vi "LIA Example Host.vi"() -> ()   [LabVIEW 2017]
uses:
  lib/host/Public/pll settings.ctl
  lib/host/Public/lock-in settings.ctl
  lib/interface/Interface/LIA Host Interface.lvclass
  lib/host/Lock-In Amplifier Example Host.lvlib
  lib/shared/Lock-In Amplifier Example Shared.lvlib
panel:
  out "Waveform Graph":cluster{"f0":dbl, "df":dbl, "magnitude":dbl[]}[](graph)
  in  "app.quit":bool
  in  "lock-in.boxcar length 0":u32=2048 caption="Boxar Length"
  in  "app.tab 0":enum32{"Lock-In", "PLL", "Output"}(tab)
  in  "lock-in.manual carrier 0":dbl=10000000.0 caption="Carrier" format="%#_6p"
  in  "lock-in.decimation 0":i32=2048 caption="Decimation" min=8 max=8192
  in  "lock-in.source 0":enum16{"AI 0", "AI 1", "AI 2", "AI 3"}(ring)=enum."AI 1" caption="Channel"
  in  "lock-in.carrier 0":T1(ring)=enum."PLL 0" caption="Carrier Source"
  in  "pll.source 0":enum16{"AI 0", "AI 1", "AI 2", "AI 3"}(ring) caption="Source"
  in  "pll.q frequency 0":dbl=10000000.0 caption="Q Frequency" format="%#_6p"
  in  "pll.reset 0":bool
  in  "ao.noise 3":dbl caption="A0 3 Noise" min=0.0 max=1.0 format="%#_6p"
  in  "ao.level 3":dbl=0.5 caption="A0 3 Level" format="%#_6pV"
  in  "ao.frequency 3":dbl=10000000.0 caption="AO 3 Frequency" format="%#.9p"
  in  "ao.frequency 0":dbl=10000000.0 caption="AO 0 Frequency" format="%#.9p"
  in  "ao.level 0":dbl=0.5 caption="AO 0 Level" format="%#_6pV"
  in  "rio device":tag="10.2.224.40" caption="Resource"
  in  "lock-in.reset boxar 0":bool
  out "lock-in.deviation 1":dbl=1.9775797561733533e-07 caption="Deviation" format="%#_6p"
  out "lock-in.amplitude 0":dbl=8.221341747482856e-05 caption="Result" format="%#_6p"
  in  "lock-in.boxcar lookback 0":i32=1024 caption="Windows to Average"
  out "Result":cluster{"mean":dbl, "trace":dbl}(graph)={"mean"=8.221341747482856e-05, "trace"=8.36741779633565e-05}
  # "NI Lock-In Amplifier Reference Example"
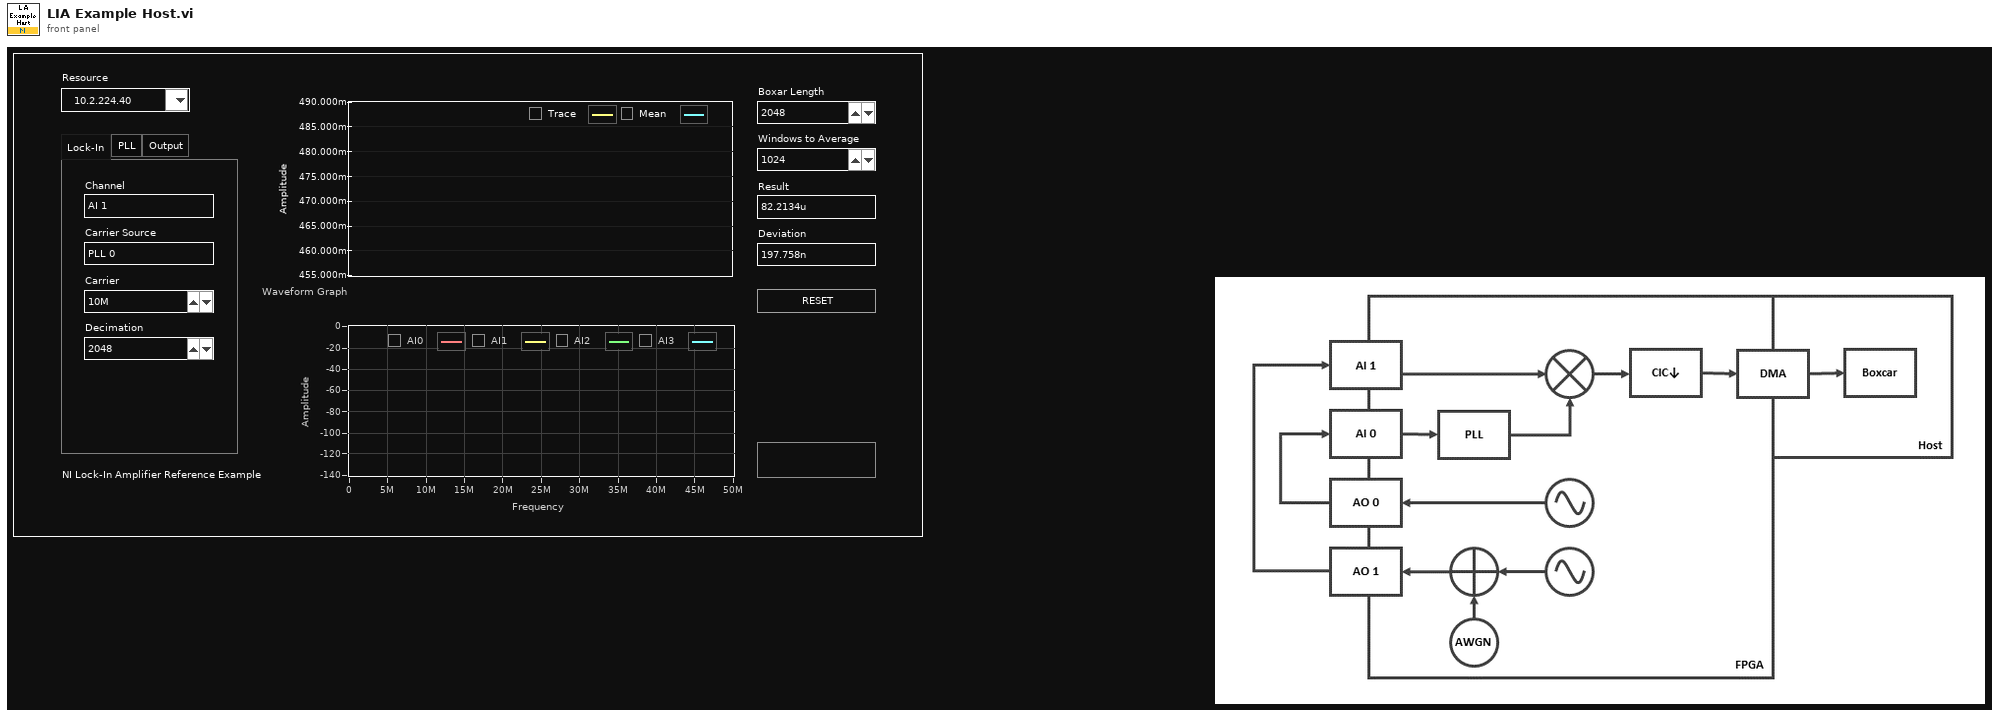
[diagram p1: front panel]
types:
  T1 = enum16{"Manual 0", "Manual 1", "Manual 2", "Manual 3", "PLL 0", "PLL 1"}
  T2 = typedef "Lock-In Amplifier Example Host.lvlib/lock-in settings.ctl" = cluster{"decimation":i32, "source":i32, "carrier source":i32, "carrier":dbl}
  T3 = typedef "Lock-In Amplifier Example Host.lvlib/pll settings.ctl" = cluster{"source":i32, "q frequency":dbl}
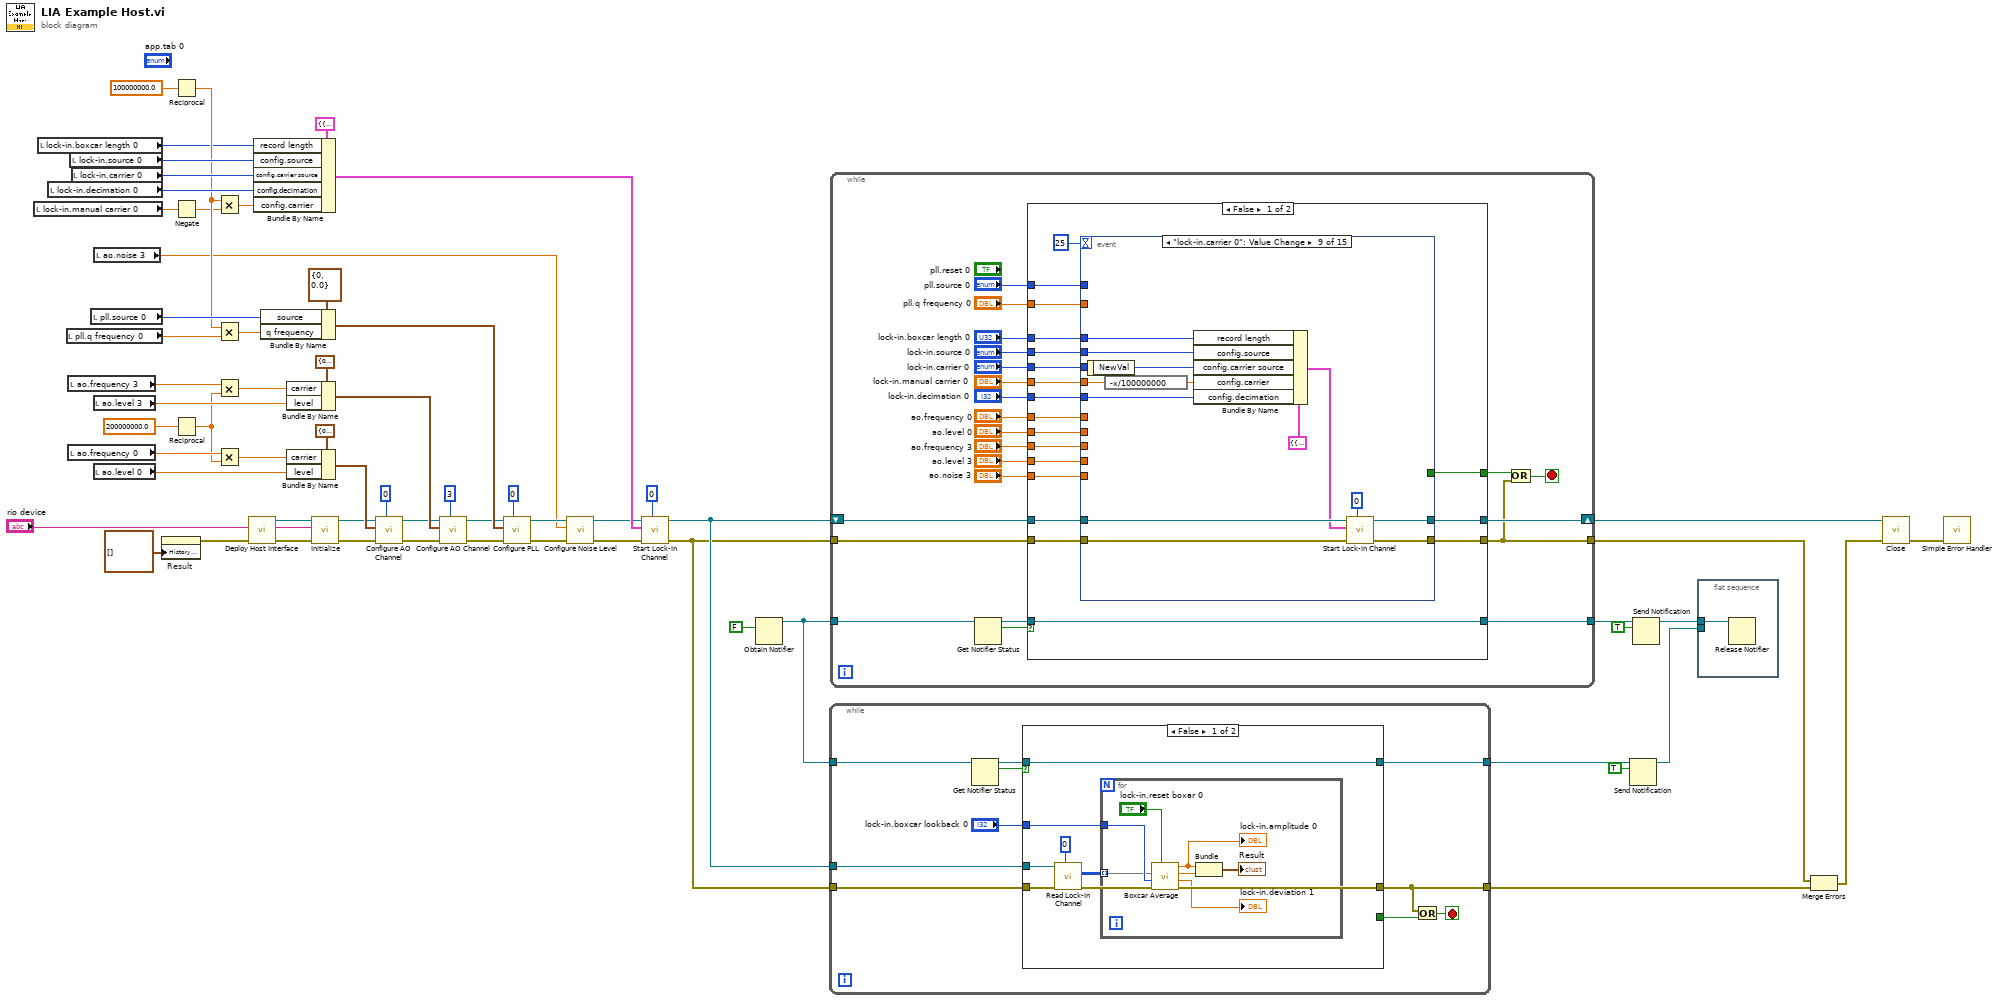
[diagram p0: block diagram]
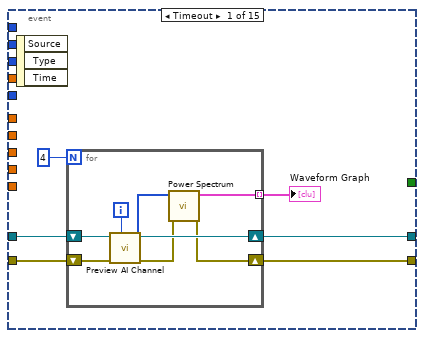
[diagram p2: hidden frame]
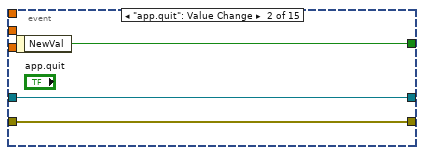
[diagram p3: hidden frame]
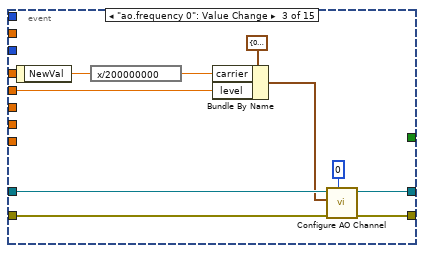
[diagram p4: hidden frame]
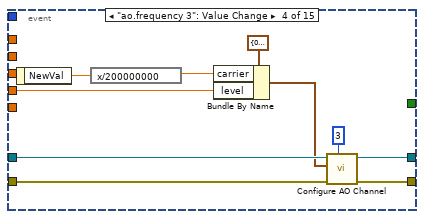
[diagram p5: hidden frame]
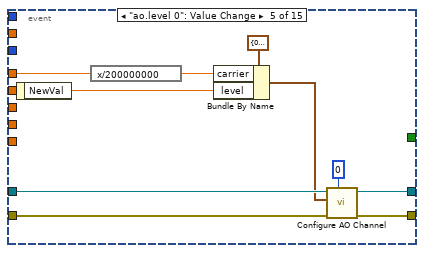
[diagram p6: hidden frame]
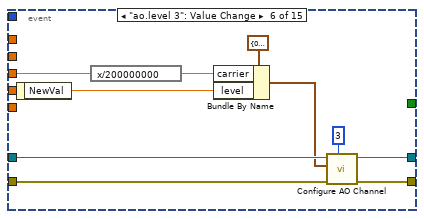
[diagram p7: hidden frame]
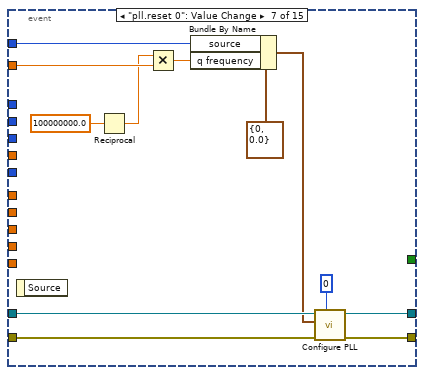
[diagram p8: hidden frame]
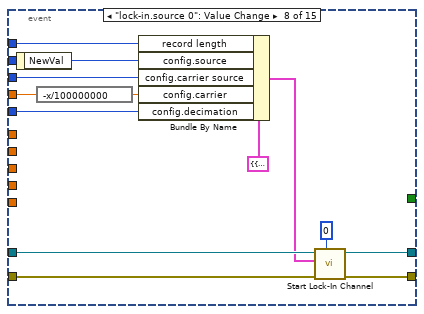
[diagram p9: hidden frame]
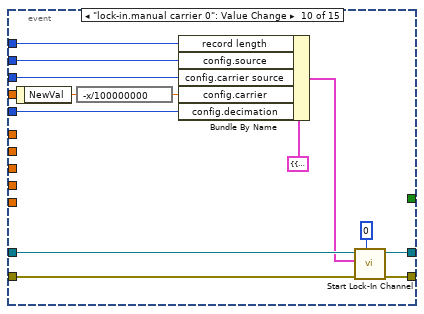
[diagram p10: hidden frame]
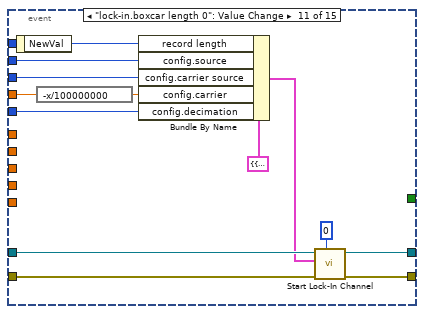
[diagram p11: hidden frame]
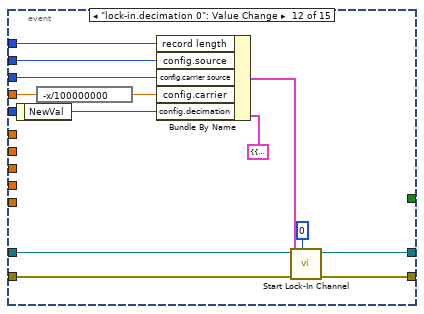
[diagram p12: hidden frame]
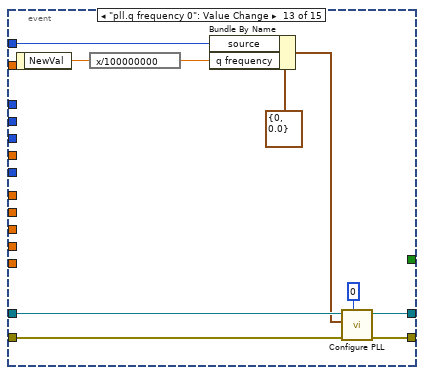
[diagram p13: hidden frame]
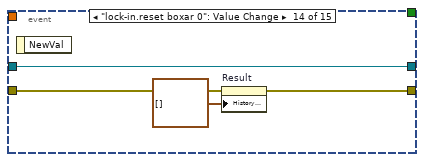
[diagram p14: hidden frame]
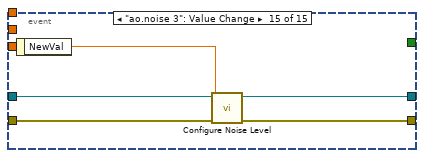
[diagram p15: hidden frame]
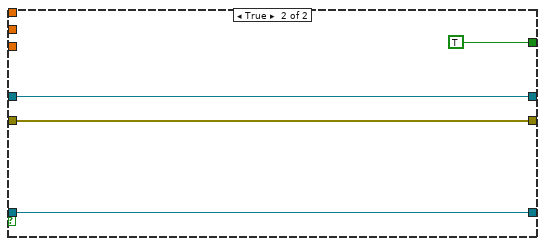
[diagram p16: hidden frame]
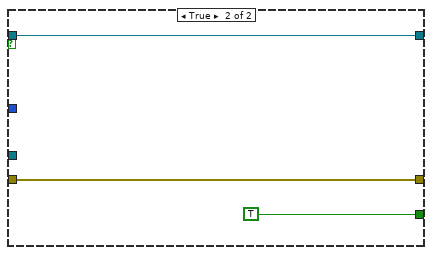
[diagram p17: hidden frame]
diagram:
  n1 = local read "lock-in.manual carrier 0"() -> (w50:dbl)
  n2 = local read "lock-in.boxcar length 0"() -> (w13:u32)
  n3 = local read "lock-in.decimation 0"() -> (w53:i32)
  n4 = local read "pll.q frequency 0"() -> (w55:dbl)
  n5 = local read "ao.frequency 3"() -> (w47:dbl)
  n6 = local read "ao.frequency 0"() -> (w44:dbl)
  n7 = local read "lock-in.source 0"() -> (w64:enum16{"AI 0", "AI 1", "AI 2", "AI 3"})
  n8 = local read "lock-in.carrier 0"() -> (w63:T1)
  n9 = local read "pll.source 0"() -> (w61:enum16{"AI 0", "AI 1", "AI 2", "AI 3"})
  n10 = local read "ao.level 3"() -> (w59:dbl)
  n11 = local read "ao.level 0"() -> (w58:dbl)
  n12 = local read "ao.noise 3"() -> (w2:dbl)
  n13 = property on="Result" class="WFChart (strict)"("History Data"=cluster{"mean":dbl, "trace":dbl}[] []) -> (error out=w8:errorcluster)  [unwired: 2 in, 1 out]
  n14 = Reciprocal(x=100000000.0) -> (1/x=w51:dbl)
  n15 = Negate(x=w50) -> (-x=w49:dbl)
  n16 = Reciprocal(x=200000000.0) -> (1/x=w43:dbl)
  n17 = Multiply(x=w51, y=w49) -> (x*y=w52:dbl)
  n18 = Multiply(x=w51, y=w55) -> (x*y=w56:dbl)
  n19 = Multiply(x=w47, y=w43) -> (x*y=w48:dbl)
  n20 = Multiply(x=w44, y=w43) -> (x*y=w45:dbl)
  n21 = call "Deploy Host Interface.vi"("error in"=w8, "resource"="rio device") -> ("error out"=w9:errorcluster, "resource out"=w10:string, "lia host interface"=w11:refnum<class "LIA Host Interface.lvclass">)  [unwired: 7 in]
  n22 = Bundle By Name(cluster=cluster{"config":T2, "record length":u32} {"config"={"decimation"=0, "source"=0, "carrier source"=0, "carrier"=0.0}, "record length"=0} ("config"), "record length"=w13, "config.source"=w64, "config.carrier source"=w63, "config.decimation"=w53, "config.carrier"=w52) -> (w14:cluster{"config":T2, "record length":u32})
  n23 = Bundle By Name(cluster=T3 {"source"=0, "q frequency"=0.0} ("config"), "source"=w61, "q frequency"=w56) -> (w40:T3)
  n24 = Bundle By Name(cluster=cluster{"carrier":dbl, "level":dbl} {"carrier"=0.0, "level"=0.0} ("config"), "carrier"=w48, "level"=w59) -> (w41:cluster{"carrier":dbl, "level":dbl})
  n25 = Bundle By Name(cluster=cluster{"carrier":dbl, "level":dbl} {"carrier"=0.0, "level"=0.0} ("config"), "carrier"=w45, "level"=w58) -> (w42:cluster{"carrier":dbl, "level":dbl})
  n26 = call-dynamic "Initialize.vi"("error in"=w9, "resource"=w10, "lia host in"=w11) -> ("error out"=w24:errorcluster, "lia host out"=w25:refnum<class "LIA Host Interface.lvclass">)  [unwired: 7 in]
  n27 = call-dynamic "Configure AO Channel.vi"("instance"=0 ("index"), "error in"=w24, "config"=w42, "lia host in"=w25) -> ("error out"=w23:errorcluster, "lia host out"=w22:refnum<class "LIA Host Interface.lvclass">)  [unwired: 6 in]
  n28 = call-dynamic "Configure AO Channel.vi"("instance"=3 ("index"), "error in"=w23, "config"=w41, "lia host in"=w22) -> ("error out"=w18:errorcluster, "lia host out"=w19:refnum<class "LIA Host Interface.lvclass">)  [unwired: 6 in]
  n29 = call-dynamic "Configure PLL.vi"("instance"=0 ("index"), "error in"=w18, "config"=w40, "lia host in"=w19) -> ("error out"=w6:errorcluster, "lia host out"=w3:refnum<class "LIA Host Interface.lvclass">)  [unwired: 6 in]
  n30 = call-dynamic "Configure Noise Level.vi"("error in"=w6, "level"=w2, "lia host in"=w3) -> ("error out"=w5:errorcluster, "lia host out"=w4:refnum<class "LIA Host Interface.lvclass">)  [unwired: 7 in]
  n31 = call-dynamic "Start Lock-In Channel.vi"("instance"=0 ("index"), "error in"=w5, "config"=w14, "lia host in"=w4) -> ("error out"=w35:errorcluster, "lia host out"=w36:refnum<class "LIA Host Interface.lvclass">)  [unwired: 6 in]
  n32 = Obtain Notifier(notification data type=FALSE) -> (notifier out=w37:refnum<notifier>)  [unwired: 3 in, 2 out]
  n33 = while {
    tunnel: w37 -> [w74]
    tunnel: w36 -> [w71]
    tunnel: w35 -> [w70]
    tunnel: [w69] -> w28
    tunnel: [w66] -> w31
    stop <- w68 stop-if-true
    n34 = Get Notifier Status(notifier=w74) -> (notifier out=w72:refnum<notifier>, current notification=w73:bool)  [unwired: 1 in, 3 out]
    n35 = case shown="False" w73 {
      tunnel: [w78 w91] -> w66
      tunnel: w72 -> [w78 w91]
      tunnel: w71 -> [w81 _]
      tunnel: w70 -> [w80 w90]
      tunnel: [w77 w90] -> w69
      tunnel: [_ TRUE] -> w67
      tunnel: "lock-in.boxcar lookback 0" -> [w76 _]
      frame False {
        n36 = call-dynamic "Read Lock-In Channel.vi"("instance"=0 ("index"), "error in"=w80, "lia host in"=w81) -> ("error out"=w77:errorcluster, "unscaled data"=w75:i64[][])  [unwired: 6 in, 1 out]
        n37 = for {
          tunnel: w75 -> [w83] mode=indexing
          tunnel: w76 -> [w84]
          n38 = call "Boxcar Average.vi"("reset"="lock-in.reset boxar 0", "sample length"=w84, "interleaved iq"=w83) -> ("standard deviation"=→"lock-in.deviation 1":dbl, "trace"=w88:dbl, "mean"=w85:dbl)  [unwired: 6 in]
          "lock-in.amplitude 0" <- w85
          n39 = Bundle("mean"=w85, "trace"=w88) -> (→"Result":cluster{"mean":dbl, "trace":dbl})  [unwired: 1 in]
        }
      }
      frame True {
      }
    }
    n40 = Or(x=w69, y=w67) -> (x .or. y?=w68:bool)
  }
  n41 = while {
    tunnel: w35 -> [w113]
    shift-right: [w99] -> w39
    shift-left: w36 -> [w112]
    tunnel: [w95] -> w27
    tunnel: w37 -> [w98]
    tunnel: [w93] -> w34
    stop <- w111 stop-if-true
    n42 = Get Notifier Status(notifier=w98) -> (notifier out=w97:refnum<notifier>, current notification=w96:bool)  [unwired: 1 in, 3 out]
    n43 = case shown="False" w96 {
      tunnel: w113 -> [w132 w288]
      tunnel: w112 -> [w131 w289]
      tunnel: [w130 w288] -> w95
      tunnel: "lock-in.manual carrier 0" -> [w128 _]
      tunnel: "lock-in.decimation 0" -> [w127 _]
      tunnel: "lock-in.source 0" -> [w126 _]
      tunnel: "lock-in.carrier 0" -> [w125 _]
      tunnel: "pll.source 0" -> [w124 _]
      tunnel: "pll.q frequency 0" -> [w123 _]
      tunnel: "ao.frequency 0" -> [w122 _]
      tunnel: "ao.level 0" -> [w121 _]
      tunnel: "ao.frequency 3" -> [w120 _]
      tunnel: "ao.level 3" -> [w119 _]
      tunnel: "ao.noise 3" -> [w118 _]
      tunnel: [w117 w289] -> w99
      tunnel: w97 -> [w115 w286]
      tunnel: [w116 TRUE] -> w94
      tunnel: [w115 w286] -> w93
      tunnel: "lock-in.boxcar length 0" -> [w114 _]
      frame False {
        n44 = event shown="[8] \"lock-in.carrier 0\": Value Change" {
          selector: _ -> [_ _ _ _ _ _ _ _ _ _ _ _ _ _ _]
          dyn-events: _ -> [_ _ _ _ _ _ _ _ _ _ _ _ _ _ _]
          timeout: 25 -> [_ _ _ _ _ _ _ _ _ _ _ _ _ _ _]
          tunnel: w132 -> [w136 w148 w154 w169 w179 w189 w201 w210 w224 w237 w249 w263 w272 w280 w284]
          tunnel: w131 -> [w137 w149 w155 w168 w178 w188 w200 w208 w222 w235 w247 w261 w271 w277 w285]
          tunnel: [w135 w148 w152 w167 w177 w187 w199 w209 w223 w236 w248 w262 w269 w279 w282] -> w130
          tunnel: w126 -> [_ _ _ _ _ _ _ _ w215 w228 w241 w257 _ _ _]
          tunnel: w125 -> [_ _ _ _ _ _ _ w213 _ w239 w252 w265 _ _ _]
          tunnel: w128 -> [_ _ _ _ _ _ _ w212 w226 _ w251 w264 _ _ _]
          tunnel: w127 -> [_ _ _ _ _ _ _ w211 w225 w238 w250 _ _ _ _]
          tunnel: w124 -> [_ _ _ _ _ _ w194 _ _ _ _ _ w274 _ _]
          tunnel: w123 -> [_ _ _ _ _ _ w195 _ _ _ _ _ _ _ _]
          tunnel: w122 -> [_ _ _ _ w172 _ _ _ _ _ _ _ _ _ _]
          tunnel: w121 -> [_ _ w157 _ _ _ _ _ _ _ _ _ _ _ _]
          tunnel: w120 -> [_ _ _ _ _ w182 _ _ _ _ _ _ _ _ _]
          tunnel: w119 -> [_ _ _ w162 _ _ _ _ _ _ _ _ _ _ _]
          tunnel: w118 -> [_ _ _ _ _ _ _ _ _ _ _ _ _ _ _]
          tunnel: [w138 w149 w150 w160 w170 w180 w190 w207 w221 w234 w246 w260 w270 w277 w283] -> w117
          tunnel: [_ w147 _ _ _ _ _ _ _ _ _ _ _ _ _] -> w116
          tunnel: w114 -> [_ _ _ _ _ _ _ w203 w218 w231 _ w255 _ _ _]
          event Timeout {
            n45 = event-data() -> ()  [unwired: 1 in, 3 out]
            n46 = for {
              N: 4 -> [_]
              shift-right: [w144] -> w138
              shift-left: w137 -> [w146]
              shift-right: [w141] -> w135
              shift-left: w136 -> [w145]
              tunnel: [w139] -> w133 mode=indexing
              i -> [w143]
              n47 = call-dynamic "Preview AI Channel.vi"("instance"=w143, "error in"=w145, "lia host in"=w146) -> ("error out"=w142:errorcluster, "samples"=w140:i16[], "lia host out"=w144:refnum<class "LIA Host Interface.lvclass">)  [unwired: 6 in]
              n48 = call "Power Spectrum.vi"("error in"=w142, "ai data"=w140) -> ("error out"=w141:errorcluster, "magnitude"=w139:cluster{"f0":dbl, "df":dbl, "magnitude":dbl[]})  [unwired: 8 in]
            }
            "Waveform Graph" <- w133
          }
          event "app.quit": Value Change {
            n49 = event-data() -> ("NewVal"=w147:bool)  [unwired: 1 in]
          }
          event "ao.frequency 0": Value Change {
            n50 = event-data() -> ("NewVal"=w156:dbl)  [unwired: 1 in]
            n51 = expression code="x/200000000"(w156) -> (w158:dbl)
            n52 = Bundle By Name(cluster=cluster{"carrier":dbl, "level":dbl} {"carrier"=0.0, "level"=0.0} ("config"), "carrier"=w158, "level"=w157) -> (w153:cluster{"carrier":dbl, "level":dbl})
            n53 = call-dynamic "Configure AO Channel.vi"("instance"=0 ("index"), "error in"=w154, "config"=w153, "lia host in"=w155) -> ("error out"=w152:errorcluster, "lia host out"=w150:refnum<class "LIA Host Interface.lvclass">)  [unwired: 6 in]
          }
          event "ao.frequency 3": Value Change {
            n54 = event-data() -> ("NewVal"=w163:dbl)  [unwired: 1 in]
            n55 = expression code="x/200000000"(w163) -> (w165:dbl)
            n56 = Bundle By Name(cluster=cluster{"carrier":dbl, "level":dbl} {"carrier"=0.0, "level"=0.0} ("config"), "carrier"=w165, "level"=w162) -> (w161:cluster{"carrier":dbl, "level":dbl})
            n57 = call-dynamic "Configure AO Channel.vi"("instance"=3 ("index"), "error in"=w169, "config"=w161, "lia host in"=w168) -> ("error out"=w167:errorcluster, "lia host out"=w160:refnum<class "LIA Host Interface.lvclass">)  [unwired: 6 in]
          }
          event "ao.level 0": Value Change {
            n58 = event-data() -> ("NewVal"=w173:dbl)  [unwired: 1 in]
            n59 = expression code="x/200000000"(w172) -> (w175:dbl)
            n60 = Bundle By Name(cluster=cluster{"carrier":dbl, "level":dbl} {"carrier"=0.0, "level"=0.0} ("config"), "carrier"=w175, "level"=w173) -> (w171:cluster{"carrier":dbl, "level":dbl})
            n61 = call-dynamic "Configure AO Channel.vi"("instance"=0 ("index"), "error in"=w179, "config"=w171, "lia host in"=w178) -> ("error out"=w177:errorcluster, "lia host out"=w170:refnum<class "LIA Host Interface.lvclass">)  [unwired: 6 in]
          }
          event "ao.level 3": Value Change {
            n62 = event-data() -> ("NewVal"=w183:dbl)  [unwired: 1 in]
            n63 = expression code="x/200000000"(w182) -> (w185:dbl)
            n64 = Bundle By Name(cluster=cluster{"carrier":dbl, "level":dbl} {"carrier"=0.0, "level"=0.0} ("config"), "carrier"=w185, "level"=w183) -> (w181:cluster{"carrier":dbl, "level":dbl})
            n65 = call-dynamic "Configure AO Channel.vi"("instance"=3 ("index"), "error in"=w189, "config"=w181, "lia host in"=w188) -> ("error out"=w187:errorcluster, "lia host out"=w180:refnum<class "LIA Host Interface.lvclass">)  [unwired: 6 in]
          }
          event "pll.reset 0": Value Change {
            n66 = event-data() -> ()  [unwired: 1 in, 1 out]
            n67 = Reciprocal(x=100000000.0) -> (1/x=w192:dbl)
            n68 = Multiply(x=w192, y=w195) -> (x*y=w197:dbl)
            n69 = Bundle By Name(cluster=T3 {"source"=0, "q frequency"=0.0} ("config"), "source"=w194, "q frequency"=w197) -> (w191:T3)
            n70 = call-dynamic "Configure PLL.vi"("instance"=0 ("index"), "error in"=w201, "config"=w191, "lia host in"=w200) -> ("error out"=w199:errorcluster, "lia host out"=w190:refnum<class "LIA Host Interface.lvclass">)  [unwired: 6 in]
          }
          event "lock-in.source 0": Value Change {
            n71 = event-data() -> ("NewVal"=w205:enum16{"AI 0", "AI 1", "AI 2", "AI 3"})  [unwired: 1 in]
            n72 = expression code="-x/100000000"(w212) -> (w214:dbl)
            n73 = Bundle By Name(cluster=cluster{"config":T2, "record length":u32} {"config"={"decimation"=0, "source"=0, "carrier source"=0, "carrier"=0.0}, "record length"=0} ("config"), "record length"=w203, "config.source"=w205, "config.carrier source"=w213, "config.carrier"=w214, "config.decimation"=w211) -> (w202:cluster{"config":T2, "record length":u32})
            n74 = call-dynamic "Start Lock-In Channel.vi"("instance"=0 ("index"), "error in"=w210, "config"=w202, "lia host in"=w208) -> ("error out"=w209:errorcluster, "lia host out"=w207:refnum<class "LIA Host Interface.lvclass">)  [unwired: 6 in]
          }
          event "lock-in.carrier 0": Value Change {
            n75 = event-data() -> ("NewVal"=w216:T1)  [unwired: 1 in]
            n76 = expression code="-x/100000000"(w226) -> (w227:dbl)
            n77 = Bundle By Name(cluster=cluster{"config":T2, "record length":u32} {"config"={"decimation"=0, "source"=0, "carrier source"=0, "carrier"=0.0}, "record length"=0} ("config"), "record length"=w218, "config.source"=w215, "config.carrier source"=w216, "config.carrier"=w227, "config.decimation"=w225) -> (w217:cluster{"config":T2, "record length":u32})
            n78 = call-dynamic "Start Lock-In Channel.vi"("instance"=0 ("index"), "error in"=w224, "config"=w217, "lia host in"=w222) -> ("error out"=w223:errorcluster, "lia host out"=w221:refnum<class "LIA Host Interface.lvclass">)  [unwired: 6 in]
          }
          event "lock-in.manual carrier 0": Value Change {
            n79 = event-data() -> ("NewVal"=w229:dbl)  [unwired: 1 in]
            n80 = expression code="-x/100000000"(w229) -> (w240:dbl)
            n81 = Bundle By Name(cluster=cluster{"config":T2, "record length":u32} {"config"={"decimation"=0, "source"=0, "carrier source"=0, "carrier"=0.0}, "record length"=0} ("config"), "record length"=w231, "config.source"=w228, "config.carrier source"=w239, "config.carrier"=w240, "config.decimation"=w238) -> (w230:cluster{"config":T2, "record length":u32})
            n82 = call-dynamic "Start Lock-In Channel.vi"("instance"=0 ("index"), "error in"=w237, "config"=w230, "lia host in"=w235) -> ("error out"=w236:errorcluster, "lia host out"=w234:refnum<class "LIA Host Interface.lvclass">)  [unwired: 6 in]
          }
          event "lock-in.boxcar length 0": Value Change {
            n83 = event-data() -> ("NewVal"=w242:u32)  [unwired: 1 in]
            n84 = expression code="-x/100000000"(w251) -> (w253:dbl)
            n85 = Bundle By Name(cluster=cluster{"config":T2, "record length":u32} {"config"={"decimation"=0, "source"=0, "carrier source"=0, "carrier"=0.0}, "record length"=0} ("config"), "record length"=w242, "config.source"=w241, "config.carrier source"=w252, "config.carrier"=w253, "config.decimation"=w250) -> (w243:cluster{"config":T2, "record length":u32})
            n86 = call-dynamic "Start Lock-In Channel.vi"("instance"=0 ("index"), "error in"=w249, "config"=w243, "lia host in"=w247) -> ("error out"=w248:errorcluster, "lia host out"=w246:refnum<class "LIA Host Interface.lvclass">)  [unwired: 6 in]
          }
          event "lock-in.decimation 0": Value Change {
            n87 = event-data() -> ("NewVal"=w258:i32)  [unwired: 1 in]
            n88 = expression code="-x/100000000"(w264) -> (w266:dbl)
            n89 = Bundle By Name(cluster=cluster{"config":T2, "record length":u32} {"config"={"decimation"=0, "source"=0, "carrier source"=0, "carrier"=0.0}, "record length"=0} ("config"), "record length"=w255, "config.source"=w257, "config.carrier source"=w265, "config.carrier"=w266, "config.decimation"=w258) -> (w254:cluster{"config":T2, "record length":u32})
            n90 = call-dynamic "Start Lock-In Channel.vi"("instance"=0 ("index"), "error in"=w263, "config"=w254, "lia host in"=w261) -> ("error out"=w262:errorcluster, "lia host out"=w260:refnum<class "LIA Host Interface.lvclass">)  [unwired: 6 in]
          }
          event "pll.q frequency 0": Value Change {
            n91 = event-data() -> ("NewVal"=w273:dbl)  [unwired: 1 in]
            n92 = expression code="x/100000000"(w273) -> (w276:dbl)
            n93 = Bundle By Name(cluster=T3 {"source"=0, "q frequency"=0.0} ("config"), "source"=w274, "q frequency"=w276) -> (w268:T3)
            n94 = call-dynamic "Configure PLL.vi"("instance"=0, "error in"=w272, "config"=w268, "lia host in"=w271) -> ("error out"=w269:errorcluster, "lia host out"=w270:refnum<class "LIA Host Interface.lvclass">)  [unwired: 6 in]
          }
          event "lock-in.reset boxar 0": Value Change {
            n95 = event-data() -> ()  [unwired: 1 in, 1 out]
            n96 = property on="Result" class="WFChart (strict)"(error in=w280, "History Data"=cluster{"mean":dbl, "trace":dbl}[] []) -> (error out=w279:errorcluster)  [unwired: 1 in, 1 out]
          }
          event "ao.noise 3": Value Change {
            n97 = event-data() -> ("NewVal"=w281:dbl)  [unwired: 1 in]
            n98 = call-dynamic "Configure Noise Level.vi"("error in"=w284, "level"=w281, "lia host in"=w285) -> ("error out"=w282:errorcluster, "lia host out"=w283:refnum<class "LIA Host Interface.lvclass">)  [unwired: 7 in]
          }
        }
      }
      frame True {
      }
    }
    n99 = Or(x=w94, y=w95) -> (x .or. y?=w111:bool)
  }
  n100 = Send Notification(notification=TRUE, notifier=w31) -> (notifier out=w29:refnum<notifier>)  [unwired: 1 in, 1 out]
  n101 = Send Notification(notification=TRUE, notifier=w34) -> (notifier out=w30:refnum<notifier>)  [unwired: 1 in, 1 out]
  n102 = flat-sequence {
    tunnel: w30 -> [w290]
    tunnel: w29 -> [_]
    frame #0 {
      n103 = Release Notifier(notifier=w290) -> ()  [unwired: 2 in, 3 out]
    }
  }
  n104 = Merge Errors(w27, w28) -> (w26:errorcluster)
  n105 = call-dynamic "Close.vi"("error in"=w26, "lia host in"=w39) -> ("error out"=w1:errorcluster)  [unwired: 8 in, 1 out]
  n106 = call <vilib>:"Simple Error Handler.vi"("error in (no error)"=w1) -> ()  [unwired: 4 in, 5 out]
